vi "Progress Bar.vi"(8 "error in (no error)":errorcluster, 11 "Label In":string) -> (0 "error out":errorcluster)   [LabVIEW 2013]
uses:
  Progress Bar Actions.ctl
panel:
  out "Progress\nLabel":string caption="Label"
  out "Label":string
  out "Progress":u8(slide) scale=0.0..100.0
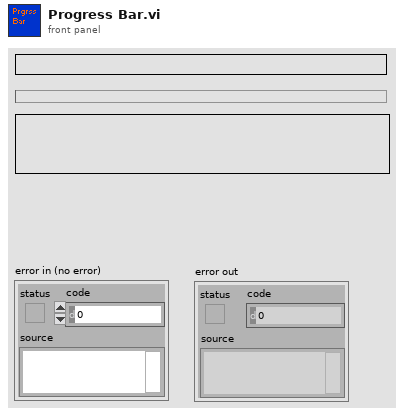
[diagram p1: front panel]
types:
  T1 = typedef "Progress Bar Actions.ctl" = enum16{"Get", "Set", "Exit", "Init"}
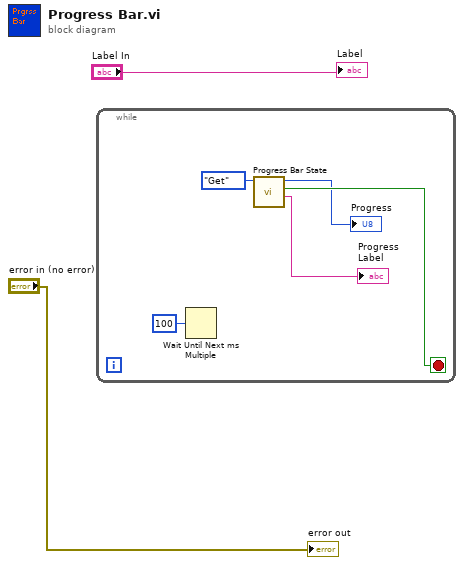
[diagram p0: block diagram]
diagram:
  n1 = while {
    stop <- w7 stop-if-true
    n2 = Wait Until Next ms Multiple(millisecond multiple=u32 100) -> ()  [unwired: 1 out]
    n3 = call "Progress Bar State.vi"("Progress Actions"=Progress_Bar_Actions."Get") -> ("String Out"=→"Progress\nLabel":string, "Exit Out"=w7:bool, "Progress Out"=→"Progress":u8)  [unwired: 3 in, 5 out]
  }
  "Label" <- "Label In"
  "error out" <- "error in (no error)"
